vi "Finish.vi"   [LabVIEW 2016]
doc: "This VI is called during exit. It can be used to close I/O refnums, save collected data, etc."
uses:
  <vilib>/Rock Robotics/Network Tables/NT Read String.vi
  <vilib>/Rock Robotics/WPI/Utilities/WPI_GetSetVariantRefNum.vi
types:
  T1 = typedef "WPI_JoystickDevRef.ctl" = cluster{"Device":T2}
  T2 = typedef "WPI_JoystickDeviceEnum.ctl" = enum16{"USB 0", "USB 1", "USB 2", "USB 3", "USB 4", "USB 5"}
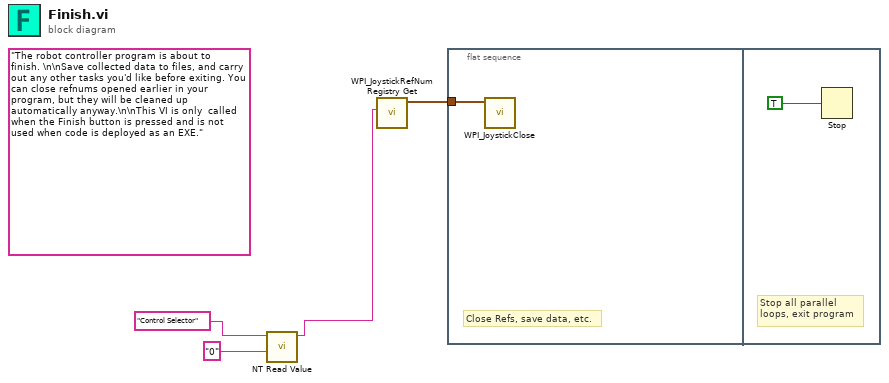
[diagram p0: block diagram]
diagram:
  (unwired) "The robot controller program is about to finish. \n\nSave collected data to files, and carry out any other tasks you'd like before exiting. You can close refnums opened earlier in your program, but they will be cleaned up automatically anyway.\n\nThis VI is only  called when the Finish button is pressed and is not used when code is deployed as an EXE."
  n1 = call-poly <vilib>:"NT Read Value.vi"("Default Value"="0", "Name"="Control Selector") -> ("String"=w1:string)  [unwired: 8 in, 1 out]
  n2 = call <vilib>:"WPI_JoystickRefNum Registry Get.vi"("refnum name"=w1) -> ("JoystickDevRef"=w4:T1)  [unwired: 1 in, 9 out]
  n3 = flat-sequence {
    tunnel: w4 -> [w5]
    frame #0 {
      # "Close Refs, save data, etc."
      n4 = call <vilib>:"WPI_JoystickClose.vi"("JoystickDevRef"=w5) -> ()  [unwired: 11 out]
    }
    frame #1 {
      # "Stop all parallel\nloops, exit program"
      n5 = Stop(stop? (T)=TRUE ("Quit")) -> ()
    }
  }
